vi "Check if configuration files exist.vi"(8 "error in (no error)":errorcluster, 11 "BMCBase in":refnum<class "BMC.lvclass">) -> (0 "error out":errorcluster, 2 "configuration file exists?":bool, 3 "BMCBase out":refnum<class "BMC.lvclass">)   [LabVIEW 2012, in "BMC.lvclass"]
doc: "Checks whether all required configuration files for the component exist."
uses:
  BMC.lvclass
  Murmex/LabVIEW/Murmex/Murmex/Murmex.lvclass
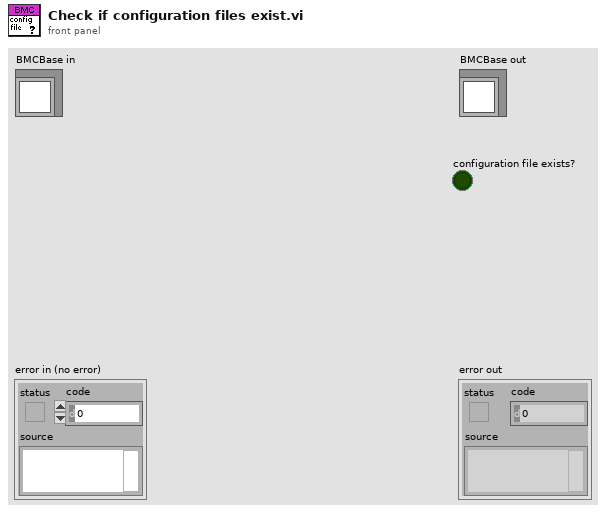
[diagram p1: front panel]
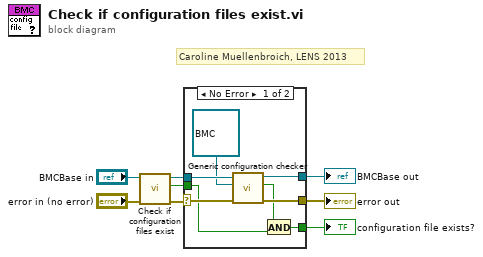
[diagram p0: block diagram]
diagram:
  # "Caroline Muellenbroich, LENS 2013"
  n1 = call-parent "Check if configuration files exist.vi"("error in (no error)"="error in (no error)", "MurmexBase in"="BMCBase in") -> ("error out"=w6:errorcluster, "configuration file exists?"=w1:bool, "MurmexBase out"=w4:refnum<class "BMC.lvclass">)  [unwired: 7 in]
  n2 = case shown="No Error" w6 {
    selector: w6 -> [w16 w18]
    tunnel: [w15 w18] -> w5
    tunnel: [w13 w17] -> w3
    tunnel: w4 -> [w14 w17]
    tunnel: [w11 _] -> w2
    tunnel: w1 -> [w9 _]
    frame No Error {
      n3 = call "Generic configuration checker.vi"("error in (no error)"=w16, "inheritance level"=refnum<class "BMC.lvclass"> refnum ("BMC"), "Murmex in"=w14) -> ("error out"=w15:errorcluster, "configuration file exists?"=w10:bool, "Murmex out"=w13:refnum<class "BMC.lvclass">)  [unwired: 6 in]
      n4 = And(x=w10, y=w9) -> (x .and. y?=w11:bool)
    }
    frame Error {
    }
  }
  "error out" <- w5
  "BMCBase out" <- w3
  "configuration file exists?" <- w2
